vi "ICR_Start_Loop.vi"(7 "Loop Selector":enum16{"OPO", "Other"}(ring), 8 "error in (no error)":errorcluster, 10 "QMH ICR Cluster":T1, 11 "QMH UI Cluster":variant) -> (0 "error out":errorcluster, 2 "Loop Current Value":i16, 3 "QMH UI Cluster Output":variant)   [LabVIEW 2024]
doc: "This VI checks if another loop is required. If yes, sends the next value to the OPO."
uses:
  controls/QMH_ICR_Cluster.ctl
  controls/HARDWARE_Resources.ctl
  controls/PROCESSING_Inputs.ctl
  controls/LOOPS_Inputs.ctl
  controls/OPO_Inputs.ctl
  controls/QMH_UI_Cluster.ctl
  controls/QMH_UI_References.ctl
  controls/QMH_UI_Report.ctl
  controls/QMH_UI_Command.ctl
  controls/QMH_ICR_Command.ctl
  controls/QMH_Status.ctl
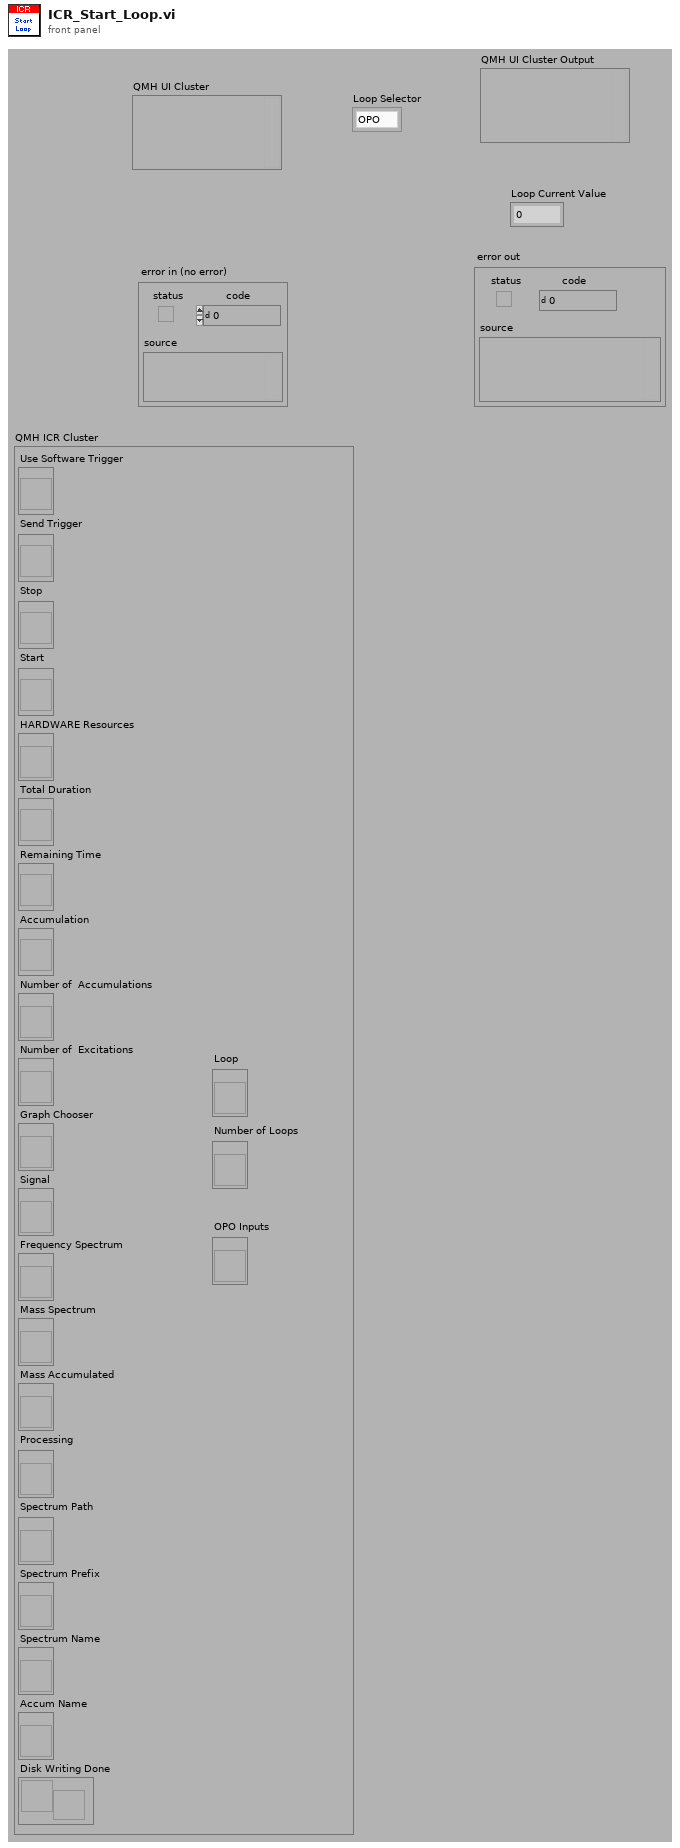
[diagram p1: front panel]
types:
  T1 = typedef "QMH_ICR_Cluster.ctl" = cluster{"Use Software Trigger":refnum<vi>, "Send Trigger":refnum<vi>, "Stop":refnum<vi>, "Start":refnum<vi>, "HARDWARE Resources":refnum<vi>, "Total Duration":refnum<vi>, "Remaining Time":refnum<vi>, "Accumulation":refnum<vi>, "Number of  Accumulations":refnum<vi>, "Number of  Excitations":refnum<vi>, "Graph Chooser":refnum<vi>, "Signal":refnum<vi>, "Frequency Spectrum":refnum<vi>, "Mass Spectrum":refnum<vi>, "Mass Accumulated":refnum<vi>, "Processing":refnum<vi>, "Spectrum Path":refnum<vi>, "Spectrum Prefix":refnum<vi>, "Spectrum Name":refnum<vi>, "Accum Name":refnum<vi>, "Disk Writing Done":refnum<notifier>, "Loop":refnum<vi>, "Number of Loops":refnum<vi>, "OPO Inputs":refnum<vi>}
  T2 = typedef "LOOPS_Inputs.ctl" = cluster{"Number of Loops":i16, "Loop Current Value":i16, "OPO Inputs":T3}
  T3 = typedef "OPO_Inputs.ctl" = cluster{"OPO AutoAlignment ON":bool, "OPO Start Value":dbl, "OPO Stop Value":dbl, "OPO Step":dbl}
  T4 = typedef "QMH_UI_Cluster.ctl" = cluster{"QMH UI References":T5, "QMH UI Report":T6}
  T5 = typedef "QMH_UI_References.ctl" = cluster{"Refnum Load":refnum<vi>, "Refnum Save As":refnum<vi>, "Refnum Start":refnum<vi>, "Refnum Exit":refnum<vi>, "Refnum Tabs":refnum<vi>, "Refnum SPECTRUM":refnum<vi>, "Refnum EXPERIMENT":refnum<vi>, "Refnum VOLTAGES":refnum<vi>, "Refnum SEQUENCE":refnum<vi>, "Refnum EXPERT":refnum<vi>, "Refnum LOOPS":refnum<vi>, "Refnum EXCIT Table":refnum<vi>, "Refnum TIMING Table":refnum<vi>, "Refnum CHANGE Experiment":refnum<vi>, "Refnum CHANGE Voltages":refnum<vi>, "Refnum CHANGE Sequence":refnum<vi>, "Refnum CHANGE Expert":refnum<vi>, "Refnum CHANGE Loops":refnum<vi>, "Refnum CHANGE Scientist":refnum<vi>, "Refnum PIL Status":refnum<vi>}
  T6 = typedef "QMH_UI_Report.ctl" = cluster{"UI Status":T7, "ICR Status":T8, "QMH Status":T9}
  T7 = typedef "QMH_UI_Command.ctl" = enum16{"Initialize", "UI Load", "UI Save", "UI Save As", "UI Change Experiment", "UI Change Voltages", "UI Change Sequence", "UI Change Expert", "UI Change Loops", "UI Change Scientist", "Ready to Start", "UI Start", "Waiting for ICR", "UI Exit", "Update Experiment", "Update Report", "Update ICR Status", "Waiting for User"}
  T8 = typedef "QMH_ICR_Command.ctl" = enum16{"Initialize", "Sequence Loop Setup", "Sequence Setup", "ICR Start", "ICR Stop", "Hardware Setup", "Next Sequence Loop", "Next Accumulation", "Waiting for Trigger", "Sequence Started", "Sequence Finished", "Sequence Loop Done", "Writing Data", "Hardware Reset", "Exit"}
  T9 = typedef "QMH_Status.ctl" = enum16{"Init", "Loading", "Setup", "Ready to Start", "Started", "Idle"}
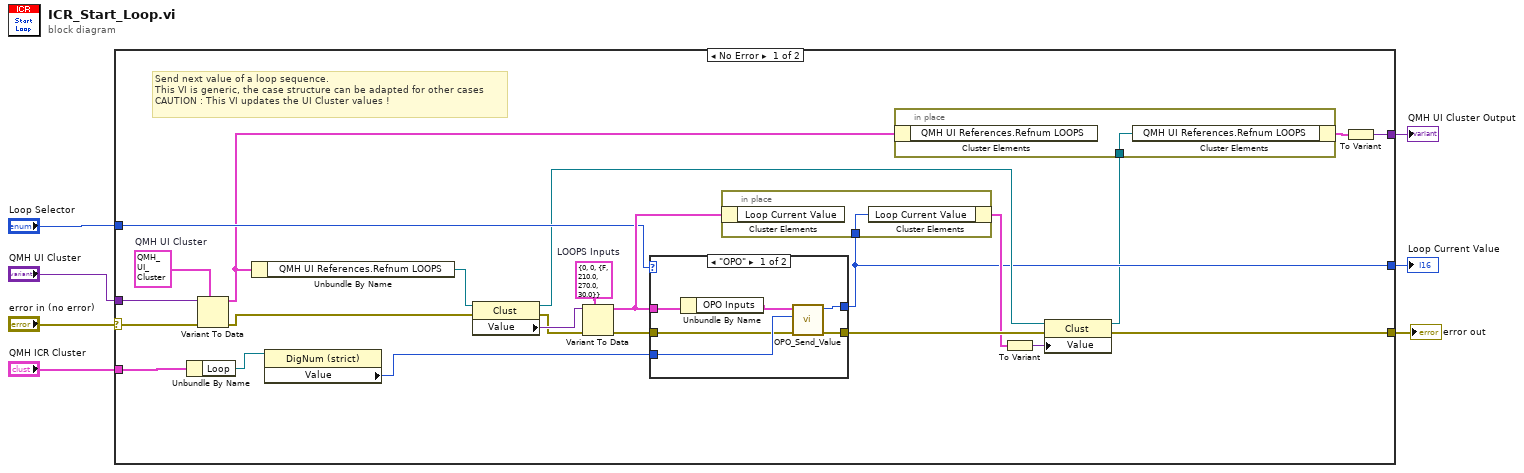
[diagram p0: block diagram]
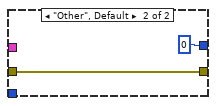
[diagram p2: hidden frame]
diagram:
  n1 = case shown="No Error" "error in (no error)" {
    selector: "error in (no error)" -> [w18 w43]
    tunnel: [w24 w43] -> w7
    tunnel: "QMH ICR Cluster" -> [w14 _]
    tunnel: "QMH UI Cluster" -> [w29 w42]
    tunnel: "Loop Selector" -> [w16 _]
    tunnel: [w12 _] -> w2
    tunnel: [w8 w42] -> w1
    frame No Error {
      w27 = T2 {"Number of Loops"=0, "Loop Current Value"=0, "OPO Inputs"={"OPO AutoAlignment ON"=FALSE, "OPO Start Value"=210.0, "OPO Stop Value"=270.0, "OPO Step"=30.0}}  # LOOPS Inputs
      w13 = T4 {"QMH UI References"={"Refnum Load"=refnum, "Refnum Save As"=refnum, "Refnum Start"=refnum, "Refnum Exit"=refnum, "Refnum Tabs"=refnum, "Refnum SPECTRUM"=refnum, "Refnum EXPERIMENT"=refnum, "Refnum VOLTAGES"=refnum, "Refnum SEQUENCE"=refnum, "Refnum EXPERT"=refnum, "Refnum LOOPS"=refnum, "Refnum EXCIT Table"=refnum, "Refnum TIMING Table"=refnum, "Refnum CHANGE Experiment"=refnum, "Refnum CHANGE Voltages"=refnum, "Refnum CHANGE Sequence"=refnum, "Refnum CHANGE Expert"=refnum, "Refnum CHANGE Loops"=refnum, "Refnum CHANGE Scientist"=refnum, "Refnum PIL Status"=refnum}, "QMH UI Report"={"UI Status"=enum."Initialize", "ICR Status"=enum."Initialize", "QMH Status"=enum."Init"}}  # QMH UI Cluster
      # "Send next value of a loop sequence.\nThis VI is generic, the case structure can be adapted for other cases\nCAUTION : This VI updates the UI Cluster values !"
      n2 = Unbundle By Name(w14) -> ("Loop"=w31:refnum<vi>)
      n3 = Variant To Data(error in=w18, type=w13, Variant=w29) -> (data=w11:T4, error out=w17:errorcluster)
      n4 = Unbundle By Name(w11) -> ("QMH UI References.Refnum LOOPS"=w30:refnum<vi>)
      n5 = property class="DigNum (strict)"(reference=w31) -> ("Value"=w26:i16)  [unwired: 1 in, 2 out]
      n6 = property class="Clust"(reference=w30, error in=w17) -> (reference out=w15:refnum<vi>, error out=w20:errorcluster, "Value"=w28:variant)
      n7 = Variant To Data(error in=w20, type=w27, Variant=w28) -> (data=w22:T2, error out=w19:errorcluster)
      n8 = case shown="\"OPO\"" w16 {
        tunnel: [w39 w40] -> w25
        tunnel: w22 -> [w36 _]
        tunnel: w26 -> [w37 _]
        tunnel: [w35 i16 0 ("OPO Value")] -> w12
        tunnel: w19 -> [w34 w40]
        frame "OPO" {
          n9 = Unbundle By Name(w36) -> ("OPO Inputs"=w38:T3)
          n10 = call "OPO_Send_Value.vi"("error in (no error)"=w34, "Loop"=w37, "OPO Inputs"=w38) -> ("error out"=w39:errorcluster, "OPO Value"=w35:i16)  [unwired: 7 in]
        }
        frame "Other", Default {
        }
      }
      n11 = in-place {
        in-place-border: w12 -> [w33]
        n12 = in-place-cluster #1(w22) -> ()  [unwired: 1 out]
        n13 = in-place-cluster #1("Loop Current Value"=w33) -> (w21:T2)
      }
      n14 = To Variant(anything=w21) -> (Variant=w23:variant)
      n15 = property class="Clust"(reference=w15, error in=w25, "Value"=w23) -> (reference out=w10:refnum<vi>, error out=w24:errorcluster)
      n16 = in-place {
        in-place-border: w10 -> [w32]
        n17 = in-place-cluster #2(w11) -> ()  [unwired: 1 out]
        n18 = in-place-cluster #2("QMH UI References.Refnum LOOPS"=w32) -> (w9:T4)
      }
      n19 = To Variant(anything=w9) -> (Variant=w8:variant)
    }
    frame Error {
    }
  }
  "error out" <- w7
  "Loop Current Value" <- w2
  "QMH UI Cluster Output" <- w1
